vi "Close.vi"(8 "error in (no error)":errorcluster, 11 "Data in":refnum<class "DAQmx - Digital Output Single Sample.lvclass">) -> (0 "error out":errorcluster, 3 "Data out":refnum<class "DAQmx - Digital Output Single Sample.lvclass">)   [LabVIEW 2021, in "DAQmx - Digital Output Single Sample.lvclass"]
doc: "Abstract Data Classes 2.1.1.13\nTim Streeter - TSA\nCopyright (c) 2025, TSA"
uses:
  DAQmx - Digital Output Single Sample.lvclass
  DAQmx - Digital Output Single Sample.lvclass/DAQmx - Digital Output Single Sample.ctl
  DAQmx-Bus.lvclass
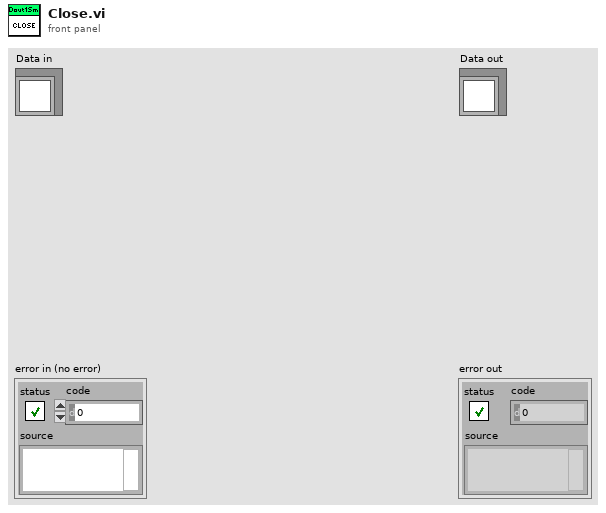
[diagram p1: front panel]
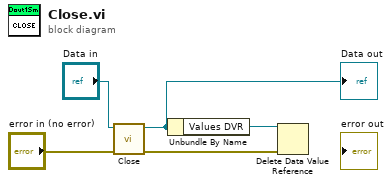
[diagram p0: block diagram]
diagram:
  n1 = call-parent "Close.vi"("error in (no error)"="error in (no error)", "Data in"="Data in") -> ("error out"=w2:errorcluster, "Data out"=w3:refnum<class "DAQmx - Digital Output Single Sample.lvclass">)  [unwired: 8 in]
  "Data out" <- w3
  n2 = Unbundle By Name(w3) -> ("Values DVR"=w1:refnum<data-value>)
  n3 = Delete Data Value Reference(data value reference=w1, error in=w2) -> ()  [unwired: 2 out]
